vi "Cash Game Live App.vi"() -> ()   [LabVIEW 2020]
panel:
  in  "Tab Control":T1(tab)
  out "Chip Stacks":dbl[][](graph)
  out "Card Map":T2(array[cluster]) {"Average Profit/Loss (BBs)" format="%#_3g"}
  out "Overall Profit/Loss (BBs)":dbl
  out "Total Hands":i32
  in  "Player":u16(ring) items=["Jonathan-M", "Mark", "Ian", "Andrew"]
  out "Card Map (Shown)":T2(array[cluster]) {"Average Profit/Loss (BBs)" format="%#_3g"}
  out "Overall Profit/Loss (BBs, Shown)":dbl
  out "Total Hands (Shown)":i32
  out "All Hands":string[](array[string])
  in  "load new":bool
  in  "reload":bool
  in  "stop":bool
  # "SUITED"
  # "OFFSUIT"
  # "A"
  # "K"
  # "Q"
  # "J"
  # "T"
  # "9"
  # "8"
  # "7"
  # "6"
  # "5"
  # "4"
  # "3"
  # "2"
  # "2"
  # "3"
  # "4"
  # "5"
  # "6"
  # "7"
  # "8"
  # "9"
  # "T"
  # "J"
  # "Q"
  # "K"
  # "A"
  # "A"
  # "K"
  # "Q"
  # "J"
  # "T"
  # "9"
  # "8"
  # "7"
  # "6"
  # "5"
  # "4"
  # "3"
  # "2"
  # "2"
  # "3"
  # "4"
  # "5"
  # "6"
  # "7"
  # "8"
  # "9"
  # "T"
  # "J"
  # "Q"
  # "K"
  # "A"
  # "SUITED"
  # "OFFSUIT"
  # "A"
  # "K"
  # "Q"
  # "J"
  # "T"
  # "9"
  # "8"
  # "7"
  # "6"
  # "5"
  # "4"
  # "3"
  # "2"
  # "2"
  # "3"
  # "4"
  # "5"
  # "6"
  # "7"
  # "8"
  # "9"
  # "T"
  # "J"
  # "Q"
  # "K"
  # "A"
  # "A"
  # "K"
  # "Q"
  # "J"
  # "T"
  # "9"
  # "8"
  # "7"
  # "6"
  # "5"
  # "4"
  # "3"
  # "2"
  # "2"
  # "3"
  # "4"
  # "5"
  # "6"
  # "7"
  # "8"
  # "9"
  # "T"
  # "J"
  # "Q"
  # "K"
  # "A"
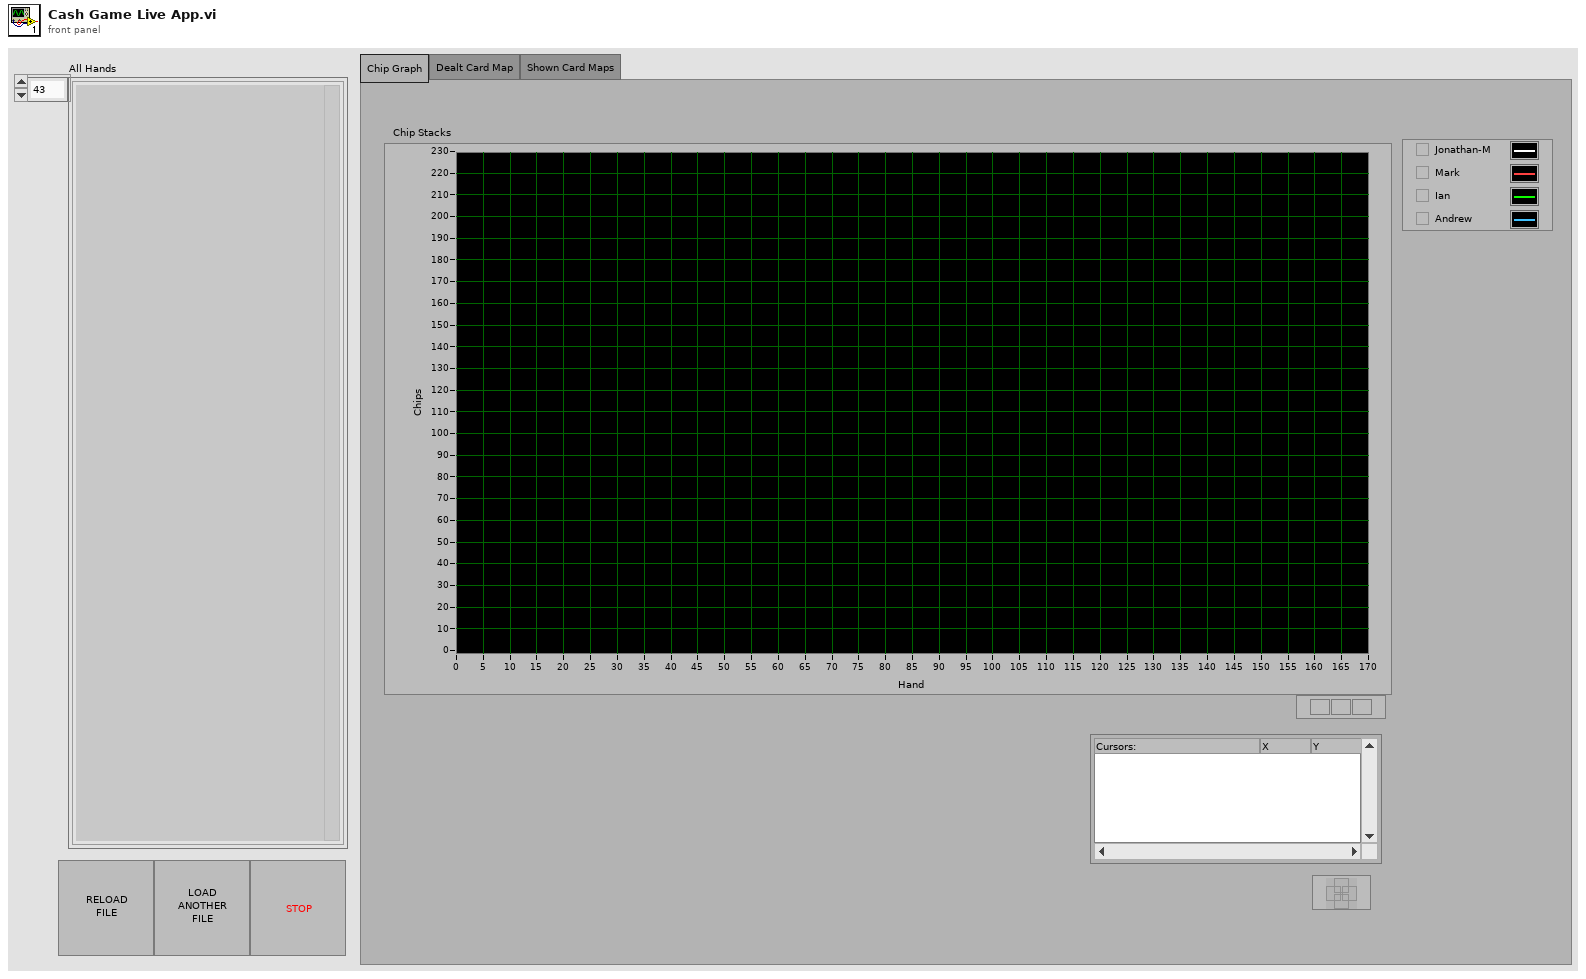
[diagram p1: front panel]
types:
  T1 = enum32{"Chip Graph", "Dealt Card Map", "Shown Card Maps"}
  T2 = cluster{"Hand Count":u16, "Average Profit/Loss (BBs)":dbl}[][]
  T3 = cluster{"Hand Count":u16, "Average Profit/Loss (BBs)":dbl}
  T4 = cluster{"Count":u16, "Profit/Loss (BBs)":dbl}[][]
  T5 = cluster{"Card Map":cluster{"Hand Count":u16, "Average Profit/Loss (BBs)":dbl}[][], "Total Hands":i32, "Overall Profit Loss (BBs)":dbl}
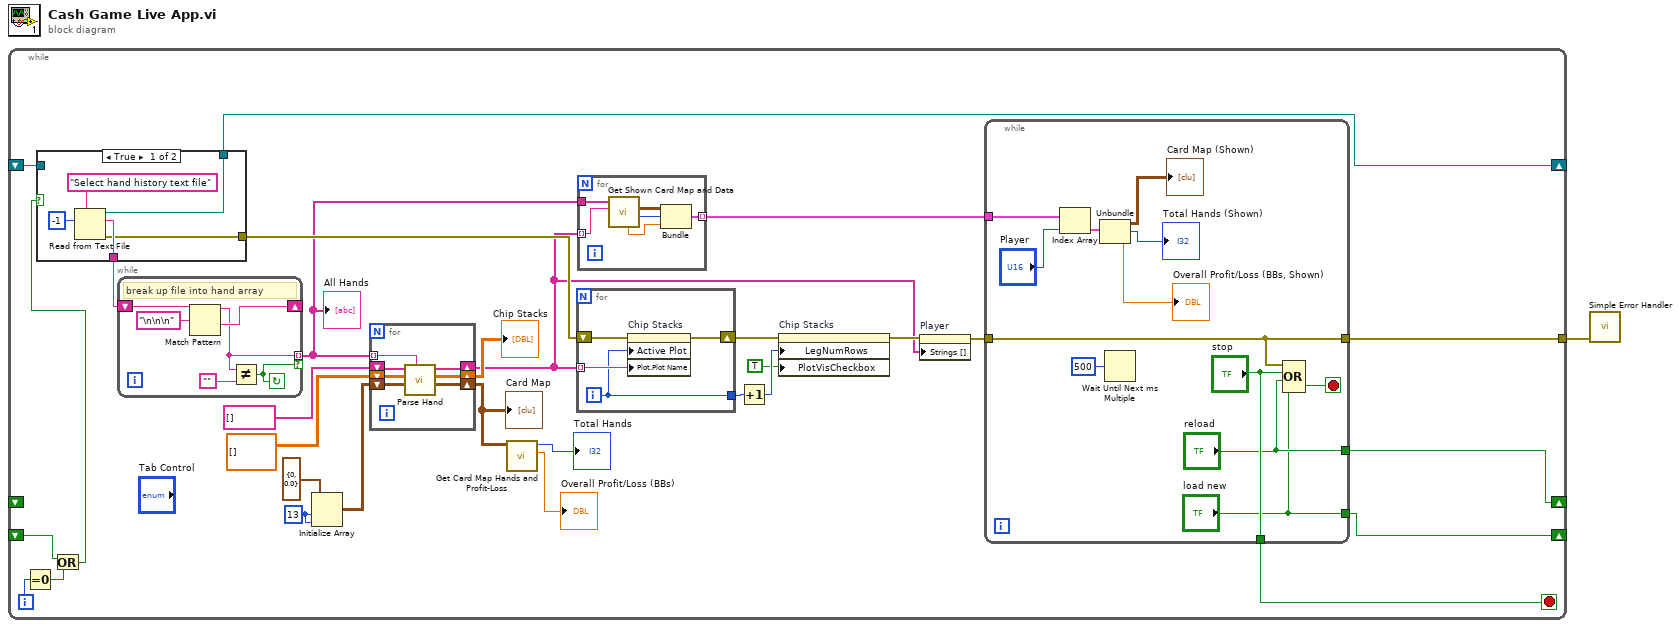
[diagram p0: block diagram]
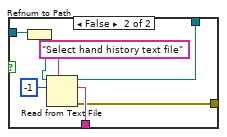
[diagram p2: hidden frame]
diagram:
  n1 = while {
    tunnel: [w10] -> w1
    shift-right: [w9] -> _
    shift-left: _ -> [w2]
    shift-right: [w8] -> _
    shift-left: _ -> [_]
    shift-right: [w7] -> _
    shift-left: _ -> [w4]
    i -> [w6]
    stop <- w11 stop-if-true
    w21 = 13 ("dimension size")
    n2 = Equal To 0?(x=w6) -> (x = 0?=w5:bool)
    n3 = Or(x=w4, y=w5) -> (x .or. y?=w3:bool)
    n4 = case shown="True" w3 {
      tunnel: [w34 w41] -> w31
      tunnel: [w33 w40] -> w29
      tunnel: [w32 w39] -> w9
      tunnel: w2 -> [_ w38]
      frame True {
        n5 = Read from Text File(prompt (Open existing file)="Select hand history text file", count=-1) -> (refnum out=w32:refnum<file>, text=w34:string, error out=w33:errorcluster)  [unwired: 2 in, 1 out]
      }
      frame False {
        n6 = Refnum to Path(1:w38) -> (0:w37:path)
        n7 = Read from Text File(prompt (Open existing file)="Select hand history text file", file (use dialog)=w37, count=-1) -> (refnum out=w39:refnum<file>, text=w41:string, error out=w40:errorcluster)  [unwired: 1 in, 1 out]
      }
    }
    n8 = while {
      shift-right: [w77] -> _
      shift-left: w31 -> [w78]
      tunnel: [w75] -> w16 mode=indexing if=w73
      stop <- w73 continue-if-true
      # "break up file into hand array"
      n9 = Match Pattern(string=w78, regular expression="\n\n\n") -> (before substring=w75:string, after substring=w77:string)  [unwired: 1 in, 2 out]
      n10 = Not Equal?(x=w75, y="") -> (x != y?=w73:bool)
    }
    "All Hands" <- w16
    n11 = Initialize Array(T3 {"Hand Count"=0, "Average Profit/Loss (BBs)"=0.0} ("Cluster"), w21, w21) -> (w20:T2)
    n12 = for {
      tunnel: w16 -> [w68] mode=indexing
      shift-right: [w71] -> w14
      shift-left: string[] [] -> [w72]
      shift-right: [w69] -> w24
      shift-left: dbl[][] [] -> [w70]
      shift-right: [w66] -> w19
      shift-left: w20 -> [w67]
      n13 = call "Parse Hand.vi"("Hand History String"=w68, "Card Map In"=w67, "Chip Stacks"=w70, "Player Names"=w72) -> ("Card Map Out"=w66:T4, "Chip Stacks Out"=w69:dbl[][], "Player Names Out"=w71:string[])  [unwired: 5 in]
    }
    "Chip Stacks" <- w24
    "Card Map" <- w19
    n14 = call "Get Card Map Hands and Profit-Loss.vi"("Card Map In"=w19) -> ("Profit/Loss (BBs)"=→"Overall Profit/Loss (BBs)":dbl, "Total Hands"=→"Total Hands":i32)  [unwired: 9 in]
    n15 = for {
      tunnel: w14 -> [w65] mode=indexing
      shift-right: [w63] -> w25
      shift-left: w29 -> [w64]
      tunnel: [w62] -> w28
      i -> [w62]
      n16 = property on="Chip Stacks" class="WFGraph (strict)"(error in=w64, "Active Plot"=w62, "Plot.Plot Name"=w65) -> (error out=w63:errorcluster)  [unwired: 1 in, 1 out]
    }
    n17 = for {
      tunnel: w16 -> [w61]
      tunnel: w14 -> [w60] mode=indexing
      tunnel: [w56] -> w12 mode=indexing
      n18 = call "Get Shown Card Map and Data.vi"("Player"=w60, "Hand Array"=w61) -> ("Total Hands"=w58:i32, "Card Map"=w59:T2, "Overall Profit Loss (BBs)"=w57:dbl)  [unwired: 6 in, 1 out]
      n19 = Bundle("Card Map"=w59, "Total Hands"=w58, "Overall Profit Loss (BBs)"=w57) -> (w56:T5)  [unwired: 1 in]
    }
    n20 = Increment(x=w28) -> (x+1=w27:i32)
    n21 = property on="Chip Stacks" class="WFGraph (strict)"(error in=w25, "LegNumRows"=w27, "PlotVisCheckbox"=TRUE ("Legend:Plot Visibility Checkbox Visible")) -> (error out=w15:errorcluster)  [unwired: 1 in, 1 out]
    n22 = property on="Player" class="Ring (strict)"(error in=w15, "Strings []"=w14) -> (error out=w13:errorcluster)  [unwired: 1 in, 1 out]
    n23 = while {
      tunnel: w13 -> [w54]
      tunnel: [w54] -> w10
      tunnel: w12 -> [w53]
      tunnel: ["stop"] -> w11
      tunnel: ["reload"] -> w8
      tunnel: ["load new"] -> w7
      stop <- w55 stop-if-true
      n24 = Index Array(array=w53, index="Player") -> (element=w51:T5)
      n25 = Unbundle(w51) -> ("Card Map"=→"Card Map (Shown)":T2, "Total Hands"=→"Total Hands (Shown)":i32, "Overall Profit Loss (BBs)"=→"Overall Profit/Loss (BBs, Shown)":dbl)
      n26 = Wait Until Next ms Multiple(millisecond multiple=u32 500) -> ()  [unwired: 1 out]
      n27 = Compound Arithmetic op=OR(w54, "stop", "reload", "load new") -> (w55:bool)
    }
  }
  n28 = call <vilib>:"Simple Error Handler.vi"("error in (no error)"=w1) -> ()  [unwired: 4 in, 5 out]
